vi "Evaluate Part 1.vi"() -> ()   [LabVIEW 2020]
uses:
  Network/Network.lvclass
panel:
  out "Steps":u64
  in  "Input":string
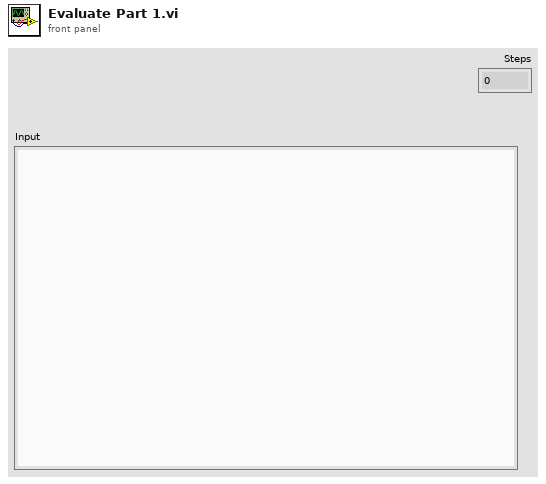
[diagram p1: front panel]
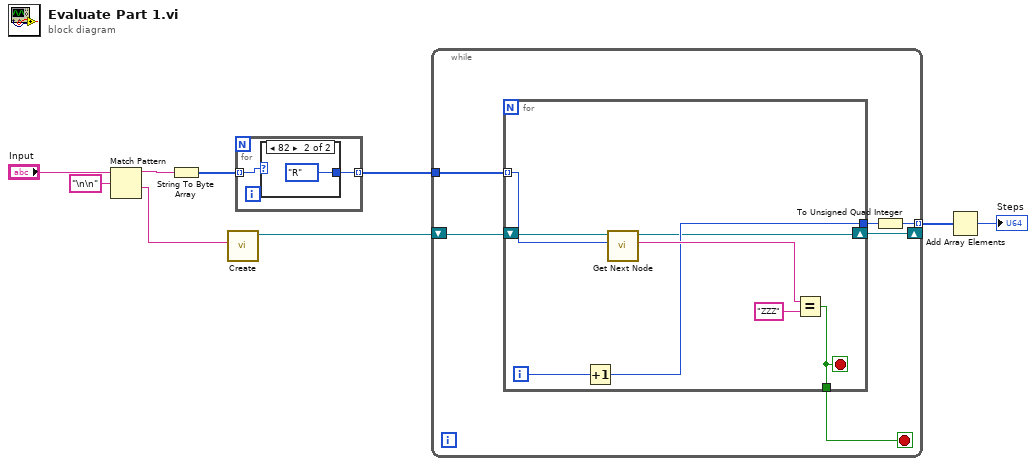
[diagram p0: block diagram]
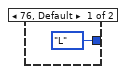
[diagram p2: hidden frame]
diagram:
  n1 = Match Pattern(string="Input", regular expression="\n\n" ("search string/char (-)")) -> (before substring=w7:string, after substring=w4:string)  [unwired: 1 in, 2 out]
  n2 = String To Byte Array(string=w7) -> (unsigned byte array=w6:u8[])
  n3 = call "Create.vi"("Input"=w4) -> ("Network"=w3:refnum<class "Network.lvclass">)  [unwired: 9 in, 1 out]
  n4 = for {
    tunnel: w6 -> [w11] mode=indexing
    tunnel: [w10] -> w5 mode=indexing
    n5 = case shown="82" w11 {
      tunnel: [enum16{"L", "R"}."L" ("Direction") enum16{"L", "R"}."R" ("Direction")] -> w10
      frame 76, Default {
      }
      frame 82 {
      }
    }
  }
  n6 = while {
    tunnel: w5 -> [w19]
    tunnel: [w14] -> w2 mode=indexing
    shift-right: [w15] -> _
    shift-left: w3 -> [w18]
    stop <- w16 stop-if-true
    n7 = for {
      tunnel: w19 -> [w26] mode=indexing
      tunnel: [w22] -> w17
      tunnel: [w21] -> w16
      shift-right: [w20] -> w15
      shift-left: w18 -> [w27]
      i -> [w23]
      stop <- w21 stop-if-true
      n8 = Increment(x=w23) -> (x+1=w22:i32)
      n9 = call "Get Next Node.vi"("Direction"=w26, "Network in"=w27) -> ("Node"=w25:string, "Network out"=w20:refnum<class "Network.lvclass">)  [unwired: 7 in, 1 out]
      n10 = Equal?(x=w25, y="ZZZ") -> (x = y?=w21:bool)
    }
    n11 = To Unsigned Quad Integer(1:w17) -> (0:w14:u64)
  }
  n12 = Add Array Elements(numeric array=w2) -> (sum=→"Steps":u64)
